vi "Test Power Supply API.vi"() -> ()   [LabVIEW 2025]
doc: "Power Supply API Tester."
uses:
  Power Supply.lvlib
  <vilib>/Utility/error.llb/DialogType.ctl
  Classes/hardware-selection.ctl
  Controls/Numeric Current.ctl
panel:
  in  "set all outputs":bool
  in  "read state":bool
  out "Numeric":dbl
  in  "read voltage":bool
  out "Amps":T1 format="%5.3f A"
  in  "read current":bool
  in  "Output Current":dbl=0.05
  in  "set current":bool
  in  "Output Voltage":dbl=10.0
  in  "set voltage":bool
  in  "Output On/Off":bool
  in  "output":bool
  in  "close":bool
  in  "init device":bool
  in  "config json file":path
  in  "read config":bool
  in  "Hardware":T2=enum."PSP-603"
  in  "select child":bool
  out "last error":errorcluster
  in  "Show Diagram on Init":bool
  in  "Run as Singleton?":bool
  in  "Show Block Diagram":bool
  in  "Refresh Modules":bool
  out "Active Modules":string[](array[string])
  in  "Stop Module":bool
  in  "Select Module":i32(ring)=-1 caption="Select Module\nTo send Request to" items=["All"=-1]
  in  "Run New Module":bool
  in  "Hide Module Panel":bool
  in  "Show Module Panel":bool
  out "Status":string
  # "This VI tests the API for the Module."
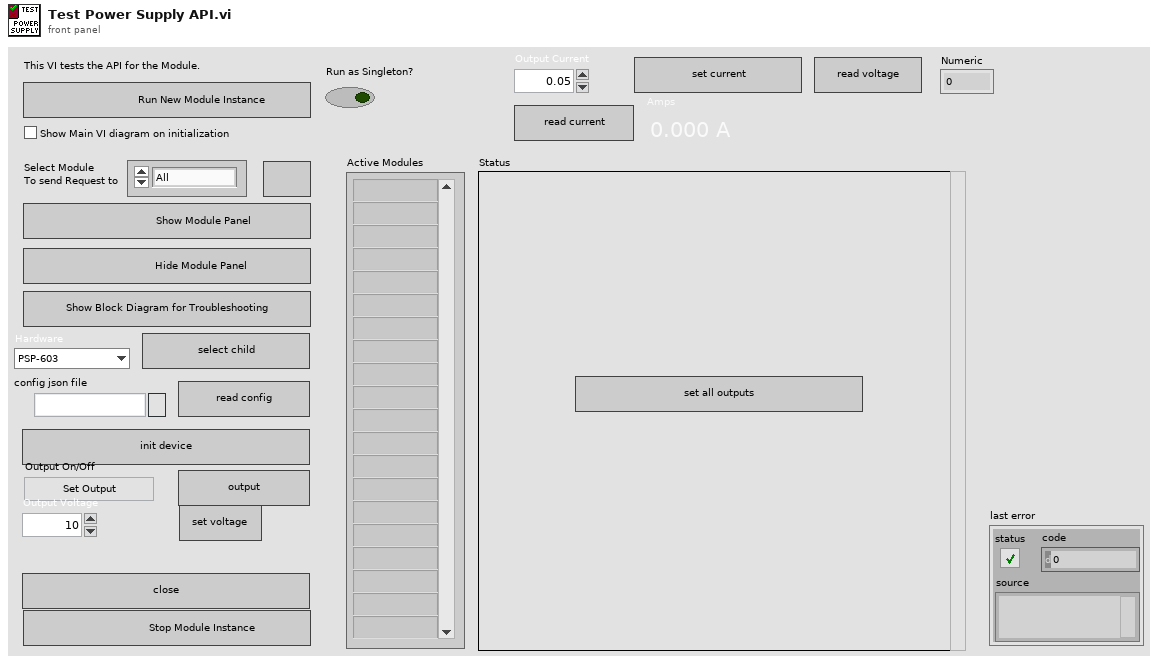
[diagram p1: front panel]
types:
  T1 = typedef "Numeric Current.ctl" = dbl
  T2 = typedef "hardware-selection.ctl" = enum16{"Parent", "Simulation", "PSP-603"}
  T3 = typedef "Power Supply.lvlib/Broadcast Events--cluster.ctl" = cluster{"Module Did Init":refnum<user-event>, "Status Updated":refnum<user-event>, "Error Reported":refnum<user-event>, "Module Did Stop":refnum<user-event>, "Update Module Execution Status":refnum<user-event>}
  T4 = typedef "DialogType.ctl" = u16
  T5 = typedef "Numeric Voltage.ctl" = dbl
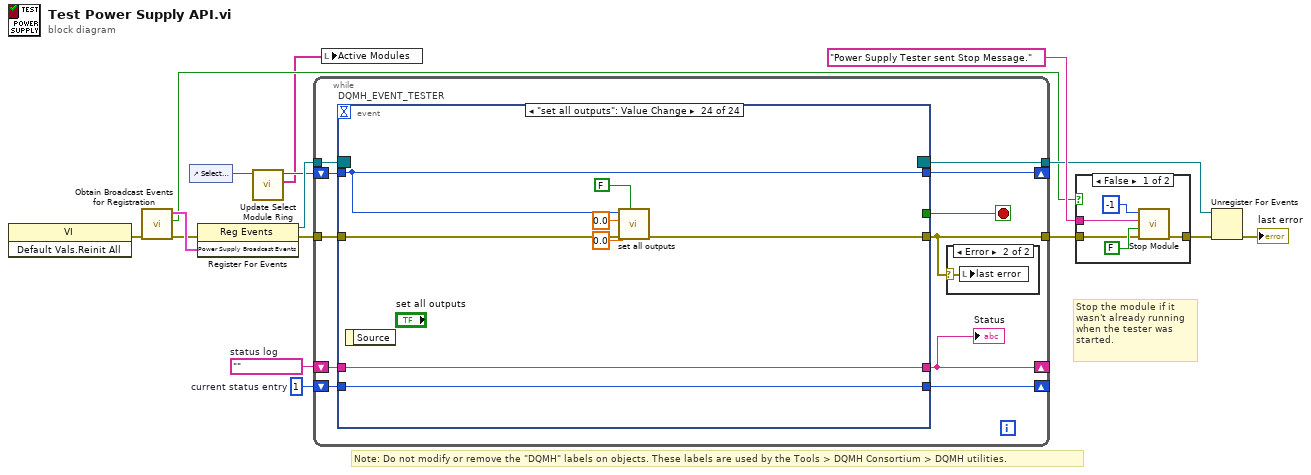
[diagram p0: block diagram]
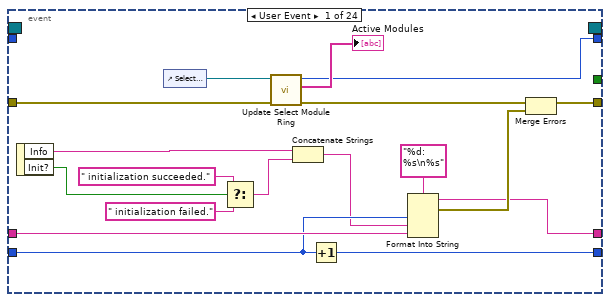
[diagram p4: hidden frame]
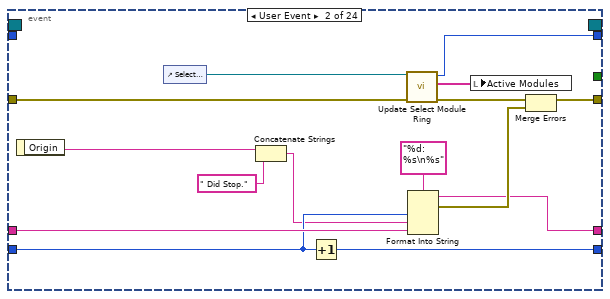
[diagram p5: hidden frame]
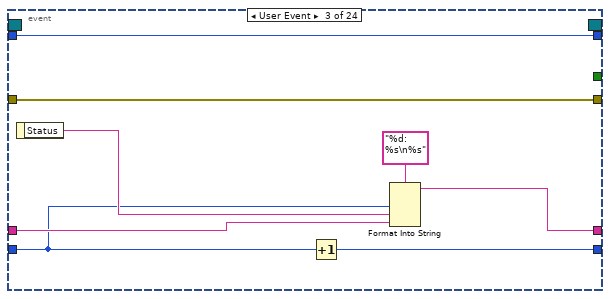
[diagram p6: hidden frame]
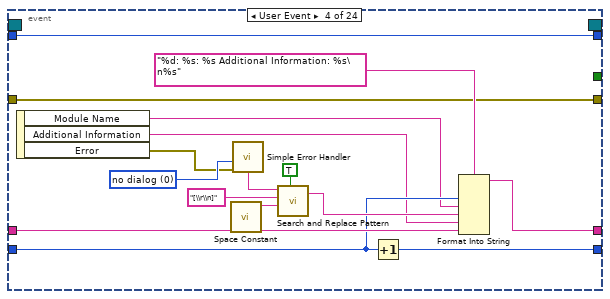
[diagram p7: hidden frame]
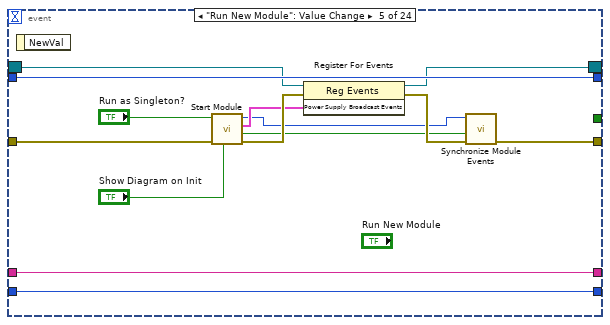
[diagram p8: hidden frame]
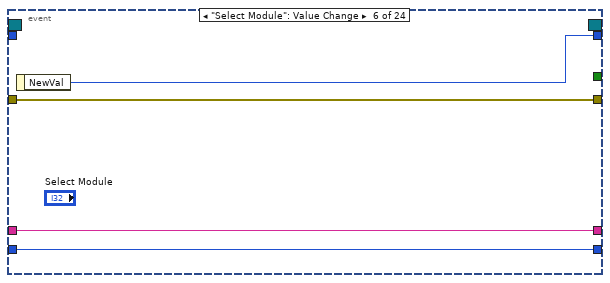
[diagram p9: hidden frame]
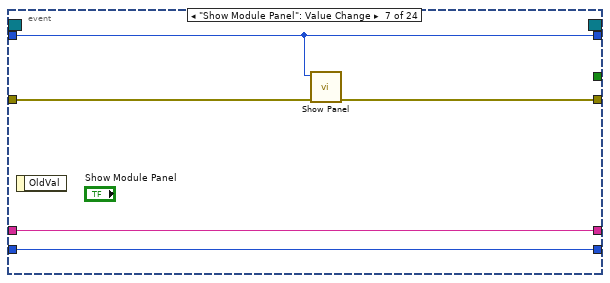
[diagram p10: hidden frame]
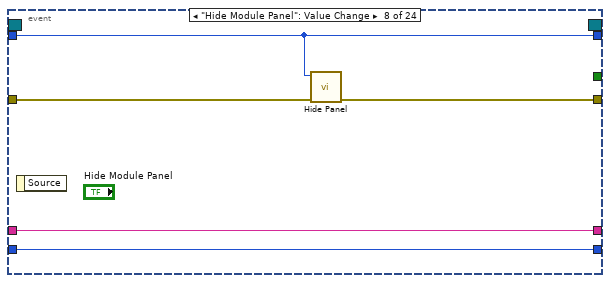
[diagram p11: hidden frame]
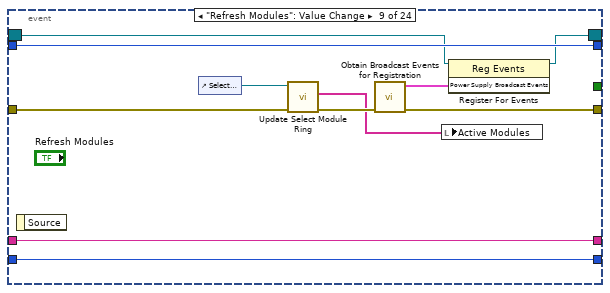
[diagram p12: hidden frame]
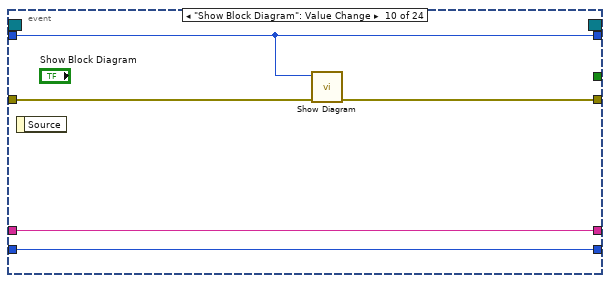
[diagram p13: hidden frame]
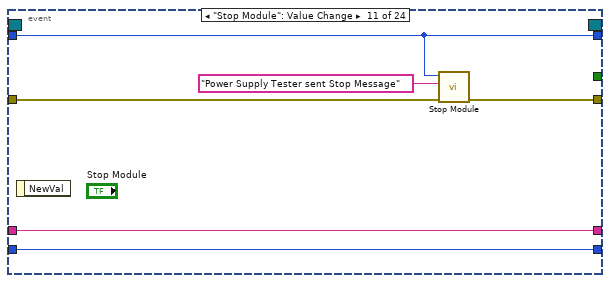
[diagram p14: hidden frame]
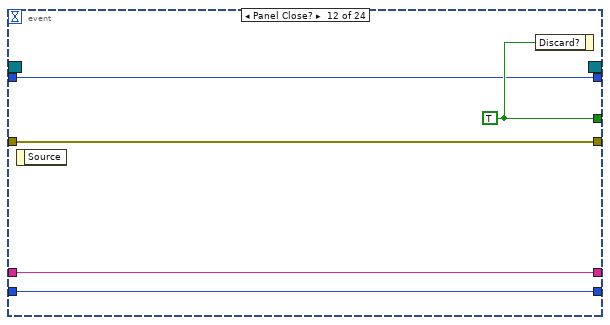
[diagram p15: hidden frame]
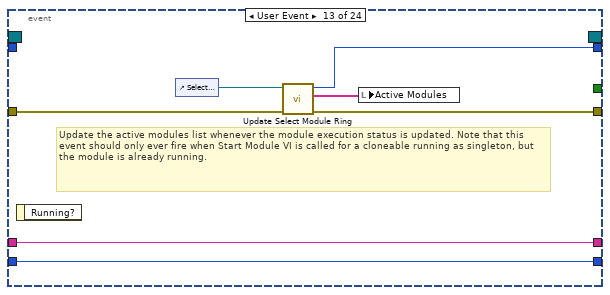
[diagram p16: hidden frame]
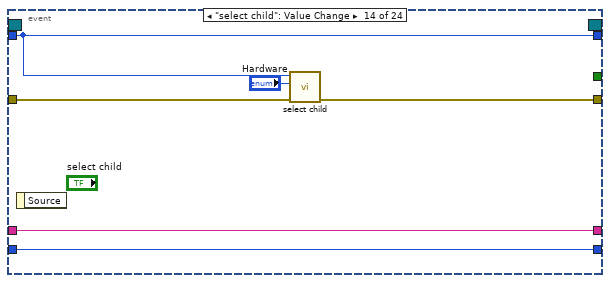
[diagram p17: hidden frame]
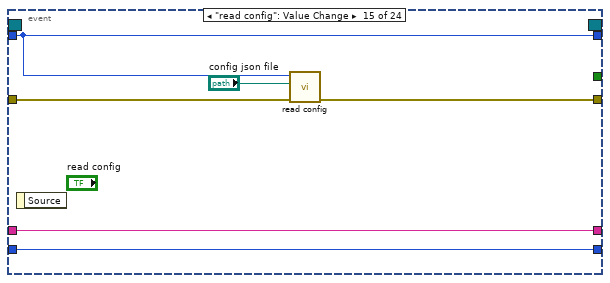
[diagram p18: hidden frame]
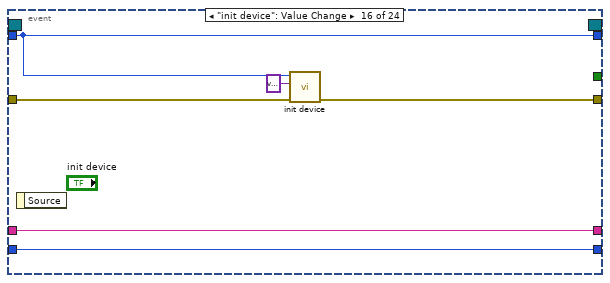
[diagram p19: hidden frame]
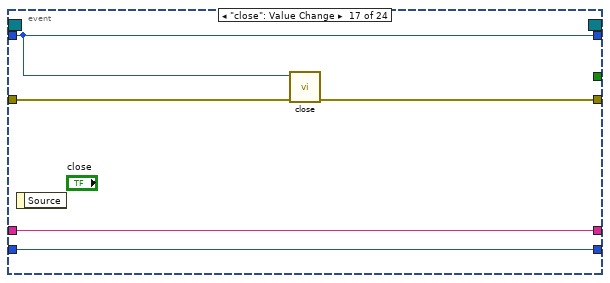
[diagram p20: hidden frame]
diagram:
  w13 = 1  # current status entry
  w14 = ""  # status log
  # "Stop the module if it wasn't already running when the tester was started."
  # "Note: Do not modify or remove the \"DQMH\" labels on objects. These labels are used by the Tools > DQMH Consortium > DQMH utilities."
  n1 = invoke class="VI" method="Default Vals.Reinit All"() -> (error out=w8:errorcluster)  [unwired: 3 in, 2 out]
  n2 = call "Obtain Broadcast Events for Registration.vi"("error in"=w8) -> ("error out"=w7:errorcluster, "Already running?"=w6:bool, "Power Supply Broadcast Events"=w12:T3)  [unwired: 8 in]
  n3 = control-ref of="Select Module"() -> (w3:refnum<vi>)
  n4 = register-events(error in=w7, w12) -> (reference out=w16:refnum<event-registration>, error out=w11:errorcluster)  [unwired: 1 in]
  n5 = call "Update Select Module Ring.vi"("Select Module Ring Ref"=w3) -> ("Active Modules (Array)"=w1:string[], "New Module Ring Value"=w2:i32)  [unwired: 8 in, 1 out]
  n6 = while {
    tunnel: w16 -> [w27]
    tunnel: [w18] -> w5
    tunnel: w11 -> [w26]
    shift-right: [w22] -> _
    shift-left: w14 -> [w24]
    shift-right: [w23] -> _
    shift-left: w13 -> [w25]
    shift-right: [w20] -> _
    shift-left: w2 -> [w21]
    tunnel: [w19] -> w9
    stop <- w17 stop-if-true
    n7 = event "DQMH_EVENT_TESTER" shown="[23] \"set all outputs\": Value Change" {
      selector: w27 -> [_ _ _ _ w93 _ _ _ w119 _ _ _ _ _ _ _ _ _ _ _ _ _ _ _]
      dyn-events: [_ _ _ _ w92 _ _ _ w118 _ _ _ _ _ _ _ _ _ _ _ _ _ _ _] -> w19
      timeout: _ -> [_ _ _ _ _ _ _ _ _ _ _ _ _ _ _ _ _ _ _ _ _ _ _ _]
      tunnel: [_ _ _ _ _ _ _ _ _ _ _ w140 _ _ _ _ _ _ _ _ _ _ _ _] -> w17
      tunnel: [w36 w53 w69 w73 w91 w103 w107 w112 w115 w126 w131 w139 w143 w149 w155 w161 w166 w172 w178 w184 w190 w196 w201 w209] -> w18
      tunnel: w26 -> [w38 w55 w69 w73 w94 w103 w108 w113 w120 w129 w132 w139 w144 w153 w159 w165 w170 w176 w182 w188 w194 w200 w205 w213]
      tunnel: w25 -> [w43 w58 w62 w76 w96 w101 w105 w110 w123 w127 w134 w137 w146 w151 w157 w163 w168 w174 w180 w186 w192 w198 w203 w211]
      tunnel: w24 -> [w44 w59 w65 w77 w97 w102 w106 w111 w124 w128 w135 w138 w147 w152 w158 w164 w169 w175 w181 w187 w193 w199 w204 w212]
      tunnel: [w41 w56 w66 w75 w97 w102 w106 w111 w124 w128 w135 w138 w147 w152 w158 w164 w169 w175 w181 w187 w193 w199 w204 w212] -> w22
      tunnel: [w42 w57 w68 w74 w96 w101 w105 w110 w123 w127 w134 w137 w146 w151 w157 w163 w168 w174 w180 w186 w192 w198 w203 w211] -> w23
      tunnel: w21 -> [_ _ w63 w85 w95 _ w104 w109 w122 w125 w133 w136 _ w150 w156 w162 w167 w173 w179 w185 w191 w197 w202 w210]
      tunnel: [w33 w50 w63 w85 w95 w100 w104 w109 w122 w125 w133 w136 w142 w150 w156 w162 w167 w173 w179 w185 w191 w197 w202 w210] -> w20
      event User Event {
        n8 = event-data() -> ("Info"=w40:string, "Init?"=w30:bool)  [unwired: 1 in]
        n9 = control-ref of="Select Module"() -> (w35:refnum<vi>)
        n10 = Select(t=" initialization succeeded.", s=w30, f=" initialization failed.") -> (s? t:f=w29:string)
        n11 = call "Update Select Module Ring.vi"("error in"=w38, "Select Module Ring Ref"=w35) -> ("error out"=w37:errorcluster, "Active Modules (Array)"=→"Active Modules":string[], "New Module Ring Value"=w33:i32)  [unwired: 7 in]
        n12 = Concatenate Strings(w40, w29) -> (w39:string)
        n13 = Increment(x=w43) -> (x+1=w42:i32)
        n14 = Format Into String(format string="%d: %s\n%s", w43, w39, w44) -> (resulting string=w41:string, error out=w46:errorcluster)  [unwired: 2 in]
        n15 = Merge Errors(w37, w46) -> (w36:errorcluster)
      }
      event User Event {
        n16 = event-data() -> ("Origin"=w48:string)  [unwired: 1 in]
        n17 = control-ref of="Select Module"() -> (w52:refnum<vi>)
        n18 = Concatenate Strings(w48, " Did Stop.") -> (w47:string)
        n19 = Increment(x=w58) -> (x+1=w57:i32)
        n20 = call "Update Select Module Ring.vi"("error in"=w55, "Select Module Ring Ref"=w52) -> ("error out"=w54:errorcluster, "Active Modules (Array)"=w51:string[], "New Module Ring Value"=w50:i32)  [unwired: 7 in]
        n21 = Format Into String(format string="%d: %s\n%s", w58, w47, w59) -> (resulting string=w56:string, error out=w61:errorcluster)  [unwired: 2 in]
        n22 = local write "Active Modules"(w51) -> ()
        n23 = Merge Errors(w54, w61) -> (w53:errorcluster)
      }
      event User Event {
        n24 = event-data() -> ("Status"=w64:string)  [unwired: 1 in]
        n25 = Increment(x=w62) -> (x+1=w68:i32)
        n26 = Format Into String(format string="%d: %s\n%s", w62, w64, w65) -> (resulting string=w66:string)  [unwired: 2 in, 1 out]
      }
      event User Event {
        w78 = T4 0 items=["no dialog", "OK message", "continue or stop message", "OK message + warnings", "continue/stop + warnings"] ("type of dialog (OK msg:1)")
        n27 = event-data() -> ("Module Name"=w72:string, "Additional Information"=w71:string, "Error"=w70:errorcluster)  [unwired: 1 in]
        n28 = call <vilib>:"Space Constant.vi"() -> ("String"=w82:string)
        n29 = call <vilib>:"Simple Error Handler.vi"("type of dialog (OK msg:1)"=w78, "error in (no error)"=w70) -> ("message"=w79:string)  [unwired: 3 in, 4 out]
        n30 = call <vilib>:"Search and Replace Pattern.vi"("string"=w79, "regular expression (\"\")"="[\\r\\n]" ("regular expression (\"\")"), "replace string (\"\")"=w82, "replace all? (F)"=TRUE ("replace all CR/LF with spaces")) -> ("result string"=w80:string)  [unwired: 1 in, 1 out]
        n31 = Increment(x=w76) -> (x+1=w74:i32)
        n32 = Format Into String(format string="%d: %s: %s Additional Information: %s\n%s", w76, w72, w80, w71, w77) -> (resulting string=w75:string)  [unwired: 2 in, 1 out]
      }
      event "Run New Module": Value Change {
        n33 = event-data() -> ()  [unwired: 1 in, 1 out]
        n34 = call "Start Module.vi"("Show Main VI Diagram on Init (F)"="Show Diagram on Init", "error in"=w94, "Run as Singleton? (F)"="Run as Singleton?") -> ("error out"=w98:errorcluster, "Wait for Event Sync?"=w90:bool, "Power Supply Broadcast Events"=w89:T3, "Module ID"=w86:i32)  [unwired: 4 in, 1 out]
        n35 = register-events(reference=w93, error in=w98, w89) -> (reference out=w92:refnum<event-registration>, error out=w99:errorcluster)
        n36 = call "Synchronize Module Events.vi"("error in"=w99, "Wait for Event Sync?"=w90, "Module ID in"=w86) -> ("error out"=w91:errorcluster)  [unwired: 7 in, 1 out]
      }
      event "Select Module": Value Change {
        n37 = event-data() -> ("NewVal"=w100:i32)  [unwired: 1 in]
      }
      event "Show Module Panel": Value Change {
        n38 = event-data() -> ()  [unwired: 1 in, 1 out]
        n39 = call "Show Panel.vi"("error in"=w108, "Module ID"=w104) -> ("error out"=w107:errorcluster)  [unwired: 9 in]
      }
      event "Hide Module Panel": Value Change {
        n40 = event-data() -> ()  [unwired: 1 in, 1 out]
        n41 = call "Hide Panel.vi"("error in"=w113, "Module ID"=w109) -> ("error out"=w112:errorcluster)  [unwired: 9 in]
      }
      event "Refresh Modules": Value Change {
        n42 = event-data() -> ()  [unwired: 1 in, 1 out]
        n43 = control-ref of="Select Module"() -> (w121:refnum<vi>)
        n44 = call "Update Select Module Ring.vi"("error in"=w120, "Select Module Ring Ref"=w121) -> ("error out"=w116:errorcluster, "Active Modules (Array)"=w114:string[])  [unwired: 7 in, 1 out]
        n45 = call "Obtain Broadcast Events for Registration.vi"("error in"=w116) -> ("error out"=w115:errorcluster, "Power Supply Broadcast Events"=w117:T3)  [unwired: 8 in, 1 out]
        n46 = local write "Active Modules"(w114) -> ()
        n47 = register-events(reference=w119, w117) -> (reference out=w118:refnum<event-registration>)  [unwired: 1 in, 1 out]
      }
      event "Show Block Diagram": Value Change {
        n48 = event-data() -> ()  [unwired: 1 in, 1 out]
        n49 = call "Show Diagram.vi"("error in"=w129, "Module ID"=w125) -> ("error out"=w126:errorcluster)  [unwired: 9 in]
      }
      event "Stop Module": Value Change {
        n50 = event-data() -> ()  [unwired: 1 in, 1 out]
        n51 = call "Stop Module.vi"("error in"=w132, "Origin"="Power Supply Tester sent Stop Message", "Module ID"=w133) -> ("error out"=w131:errorcluster)  [unwired: 8 in]
      }
      event Panel Close? {
        w140 = TRUE ("Discard?")
        n52 = event-data() -> ()  [unwired: 1 in, 1 out]
        n53 = event-data("Discard?"=w140) -> ()  [unwired: 1 in, 1 out]
      }
      event User Event {
        # "Update the active modules list whenever the module execution status is updated. Note that this event should only ever fire when Start Module VI is called for a cloneable running as singleton, but the module is already running."
        n54 = event-data() -> ()  [unwired: 1 in, 1 out]
        n55 = control-ref of="Select Module"() -> (w145:refnum<vi>)
        n56 = call "Update Select Module Ring.vi"("error in"=w144, "Select Module Ring Ref"=w145) -> ("error out"=w143:errorcluster, "Active Modules (Array)"=w141:string[], "New Module Ring Value"=w142:i32)  [unwired: 7 in]
        n57 = local write "Active Modules"(w141) -> ()
      }
      event "select child": Value Change {
        n58 = event-data() -> ()  [unwired: 1 in, 1 out]
        n59 = call "select child.vi"("error in"=w153, "Enum"="Hardware", "Module ID"=w150) -> ("error out"=w149:errorcluster)  [unwired: 7 in, 1 out]
      }
      event "read config": Value Change {
        n60 = event-data() -> ()  [unwired: 1 in, 1 out]
        n61 = call "read config.vi"("error in"=w159, "config json file"="config json file", "Module ID"=w156) -> ("error out"=w155:errorcluster)  [unwired: 7 in, 1 out]
      }
      event "init device": Value Change {
        n62 = event-data() -> ()  [unwired: 1 in, 1 out]
        n63 = call "init device.vi"("error in"=w165, "Variant"=variant, "Module ID"=w162) -> ("error out"=w161:errorcluster)  [unwired: 7 in, 1 out]
      }
      event "close": Value Change {
        n64 = event-data() -> ()  [unwired: 1 in, 1 out]
        n65 = call "close.vi"("error in"=w170, "Module ID"=w167) -> ("error out"=w166:errorcluster)  [unwired: 8 in, 1 out]
      }
      event "output": Value Change {
        n66 = event-data() -> ()  [unwired: 1 in, 1 out]
        n67 = call "output.vi"("error in"=w176, "Output On/Off"="Output On/Off", "Module ID"=w173) -> ("error out"=w172:errorcluster)  [unwired: 7 in, 1 out]
      }
      event "set voltage": Value Change {
        n68 = event-data() -> ()  [unwired: 1 in, 1 out]
        n69 = call "set voltage.vi"("error in"=w182, "Output Voltage"="Output Voltage", "Module ID"=w179) -> ("error out"=w178:errorcluster)  [unwired: 7 in, 1 out]
      }
      event "set current": Value Change {
        n70 = event-data() -> ()  [unwired: 1 in, 1 out]
        n71 = call "set current.vi"("error in"=w188, "Output Current"="Output Current", "Module ID"=w185) -> ("error out"=w184:errorcluster)  [unwired: 7 in, 1 out]
      }
      event "read current": Value Change {
        n72 = event-data() -> ()  [unwired: 1 in, 1 out]
        n73 = call "read current.vi"("error in"=w194, "Module ID"=w191) -> ("error out"=w190:errorcluster, "Amps"=→"Amps":T1)  [unwired: 7 in, 1 out]
      }
      event "read voltage": Value Change {
        n74 = event-data() -> ()  [unwired: 1 in, 1 out]
        n75 = call "read voltage.vi"("error in"=w200, "Module ID"=w197) -> ("error out"=w196:errorcluster, "Volts"=→"Numeric":T5)  [unwired: 7 in, 1 out]
      }
      event "read state": Value Change {
        n76 = event-data() -> ()  [unwired: 1 in, 1 out]
        n77 = call "read state.vi"("error in"=w205, "Module ID"=w202) -> ("error out"=w201:errorcluster)  [unwired: 7 in, 2 out]
      }
      event "set all outputs": Value Change {
        n78 = event-data() -> ()  [unwired: 1 in, 1 out]
        n79 = call "set all outputs.vi"("Output On/Off"=FALSE, "error in"=w213, "Current"=0.0, "Voltage"=0.0, "Module ID"=w210) -> ("error out"=w209:errorcluster)  [unwired: 5 in, 1 out]
      }
    }
    "Status" <- w22
    n80 = case shown="Error" w18 {
      selector: w18 -> [_ w28]
      frame No Error {
      }
      frame Error {
        n81 = local write "last error"(w28) -> ()
      }
    }
  }
  n82 = local write "Active Modules"(w1) -> ()
  n83 = case shown="False" w6 {
    tunnel: [w218 w219] -> w15
    tunnel: "Power Supply Tester sent Stop Message." ("Origin") -> [w217 _]
    tunnel: w5 -> [w214 w219]
    frame False {
      n84 = call "Stop Module.vi"("error in"=w214, "Wait for Module to stop? (F)"=FALSE ("Wait for Module to stop?"), "Origin"=w217, "Module ID"=-1 ("Stop all")) -> ("error out"=w218:errorcluster)  [unwired: 7 in]
    }
    frame True {
    }
  }
  n85 = Unregister For Events(event registration refnum=w9, error in=w15) -> (error out=→"last error":errorcluster)
